vi "Copy Between Trees.vi"() -> ()   [LabVIEW 2021, in "Tree Map.lvlib"]
doc: "<b>Author:</b> Piotr Kruczkowski <PrimaryKey>\n<b>License:</b> NewBSD\n\nCopyright (c) 2019, National Instruments\nAll rights reserved.\n\nRedistribution and use in source and binary forms, with or without\nmodification, are permitted provided that the following conditions are met:\n1. Redistributions of source code must retain the above copyright\n notice, this list of conditions and the following disclaimer.\n2. Redistributions in binary form must reproduce the above copyright\n notice, this list of conditions and the following disclaimer in the\n documentation and/or other materials provided with the distribution.\n3. Neither the name of National Instruments nor the\n names of its contributors may be used to endorse or promote products\n derived from this software without specific prior written permission.\n\nTHIS SOFTWARE IS PROVIDED BY National Instruments ''AS IS'' AND ANY\nEXPRESS OR IMPLIED WARRANTIES, INCLUDING, BUT NOT LIMITED TO, THE IMPLIED\nWARRANTIES OF MERCHANTABILITY AND FITNESS FOR A PARTICULAR PURPOSE ARE\nDISCLAIMED. IN NO EVENT SHALL National Instruments BE LIABLE FOR ANY\nDIRECT, INDIRECT, INCIDENTAL, SPECIAL, EXEMPLARY, OR CONSEQUENTIAL DAMAGES\n(INCLUDING, BUT NOT LIMITED TO, PROCUREMENT OF SUBSTITUTE GOODS OR SERVICES;\nLOSS OF USE, DATA, OR PROFITS; OR BUSINESS INTERRUPTION) HOWEVER CAUSED AND\nON ANY THEORY OF LIABILITY, WHETHER IN CONTRACT, STRICT LIABILITY, OR TORT\n(INCLUDING NEGLIGENCE OR OTHERWISE) ARISING IN ANY WAY OUT OF THE USE OF THIS\nSOFTWARE, EVEN IF ADVISED OF THE POSSIBILITY OF SUCH DAMAGE."
uses:
  <vilib>/National Instruments/Tree Map/Tree Map.lvlib
  <vilib>/National Instruments/Tree Map/API/List Roots.vi
  <vilib>/National Instruments/Tree Map/Utility/Into Tree Control Items.vi
panel:
  out "New Paths":set{string}(c389)={"\\BaseTree\\System\\SubSystem", "\\BaseTree\\System\\SubSystem\\NestedNode"}
  in  "Tree Control":string(tree)
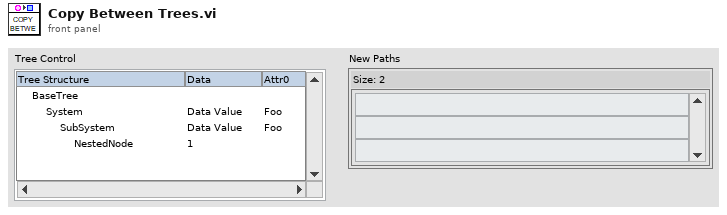
[diagram p1: front panel]
types:
  T1 = typedef "Tree Map.lvlib/Tree Map Data.ctl" = map{string, cluster{"Child Paths Set":set{string}, "Name":string, "Data":string, "Attributes":map{string, string}}}
  T2 = cluster{"Left Cell String":string, "Child Text":string[], "Child Tag":string, "Item Indent":i32, "Child Only?":bool, "Glyph Index":i32}[]
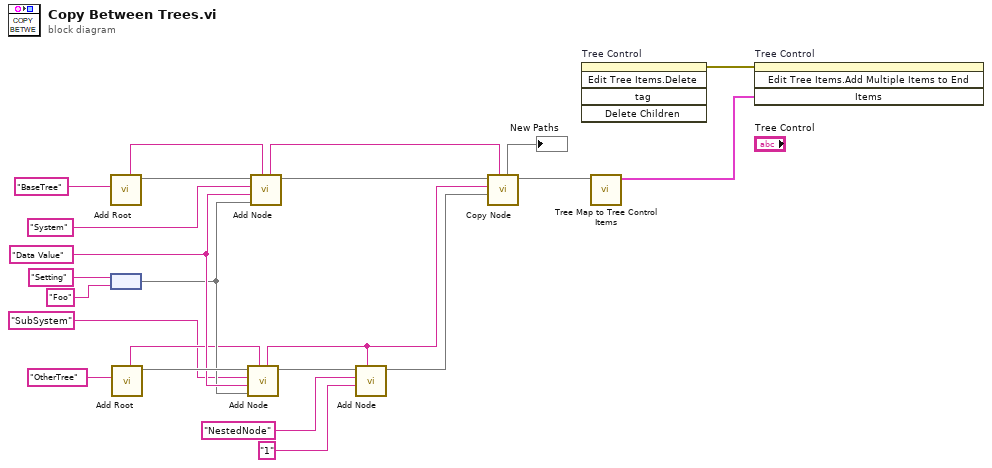
[diagram p0: block diagram]
diagram:
  w11 = "Data Value" ("New Root Name")
  n1 = call <vilib>:"Add Root.vi"("New Root Name"="BaseTree") -> ("Tree Map Out"=w21:T1, "Root Path"=w17:string)  [unwired: 9 in]
  n2 = node("Setting" ("New Root Name"), "Foo" ("New Root Name")) -> (w10:map{string, string})
  n3 = call <vilib>:"Add Root.vi"("New Root Name"="OtherTree") -> ("Tree Map Out"=w13:T1, "Root Path"=w9:string)  [unwired: 9 in]
  n4 = call <vilib>:"Add Node.vi"("Parent Path"=w9, "Attributes"=w10, "Data"=w11, "New Node Name"="SubSystem" ("New Root Name"), "Tree Map In"=w13) -> ("Tree Map Out"=w6:T1, "New Node Path"=w3:string)  [unwired: 4 in, 1 out]
  n5 = call <vilib>:"Add Node.vi"("Parent Path"=w17, "Attributes"=w10, "Data"=w11, "New Node Name"="System" ("New Root Name"), "Tree Map In"=w21) -> ("Tree Map Out"=w20:T1, "New Node Path"=w8:string)  [unwired: 4 in, 1 out]
  n6 = call <vilib>:"Add Node.vi"("Parent Path"=w3, "Data"="1" ("New Node Name"), "New Node Name"="NestedNode", "Tree Map In"=w6) -> ("Tree Map Out"=w5:T1)  [unwired: 5 in, 2 out]
  n7 = call <vilib>:"Copy Node.vi"("New Parent Path in Target"=w8, "Source Tree Map (Use Target)"=w5, "Node Path in Source"=w3, "Target Tree Map In"=w20) -> ("Target Tree Map Out"=w15:T1, "New Paths"=→"New Paths":set{string})  [unwired: 5 in, 1 out]
  n8 = invoke on="Tree Control" class="Tree (strict)" method="Edit Tree Items.Delete"() -> (error out=w23:errorcluster)  [unwired: 5 in, 4 out]
  n9 = call <vilib>:"Tree Map to Tree Control Items.vi"("Tree Map In"=w15) -> ("Tree Control Items"=w16:T2)  [unwired: 10 in]
  n10 = invoke on="Tree Control" class="Tree (strict)" method="Edit Tree Items.Add Multiple Items to End"(error in=w23, "Items"=w16) -> ()  [unwired: 2 in, 4 out]
